vi "Timer (SubVI).vi"(1 "Stop":bool) -> (0 "T":dbl)   [LabVIEW 2011]
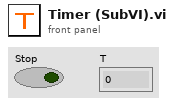
[diagram p1: front panel]
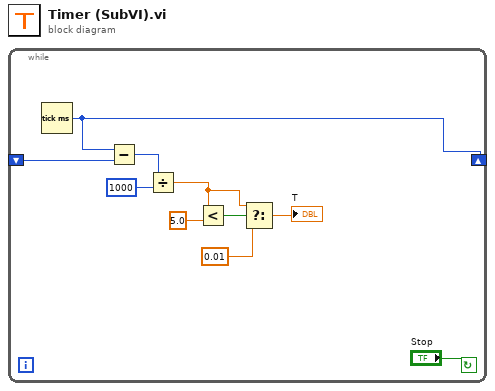
[diagram p0: block diagram]
diagram:
  n1 = while {
    shift-right: [w10] -> _
    shift-left: _ -> [w9]
    stop <- "Stop" continue-if-true
    n2 = Tick Count (ms)() -> (millisecond timer value=w10:u32)
    n3 = Subtract(x=w10, y=w9) -> (x-y=w8:u32)
    n4 = Divide(x=w8, y=u32 1000) -> (x/y=w4:dbl)
    n5 = Less?(x=w4, y=5.0) -> (x < y?=w5:bool)
    n6 = Select(t=w4, s=w5, f=0.01) -> (s? t:f=→"T":dbl)
  }
